vi "Periodic Step Down.vi"(8 "error in (no error)":errorcluster caption="entrée d'erreur (pas d'erreur)", 11 "Game Board en entrée":refnum<class "Game Board.lvclass">) -> (0 "error out":errorcluster caption="sortie d'erreur", 2 "Freeze Piece":bool, 3 "Game Board en sortie":refnum<class "Game Board.lvclass">)   [LabVIEW 2017, in "Game Board.lvclass"]
uses:
  Game Board.lvclass
  Controls/Moves.ctl
  Controls/Coordinates.ctl
  Game Board.lvclass/Game Board.ctl
  Piece of Bricks_class/Piece of Bricks.lvclass
  Wall_class/Wall.lvclass
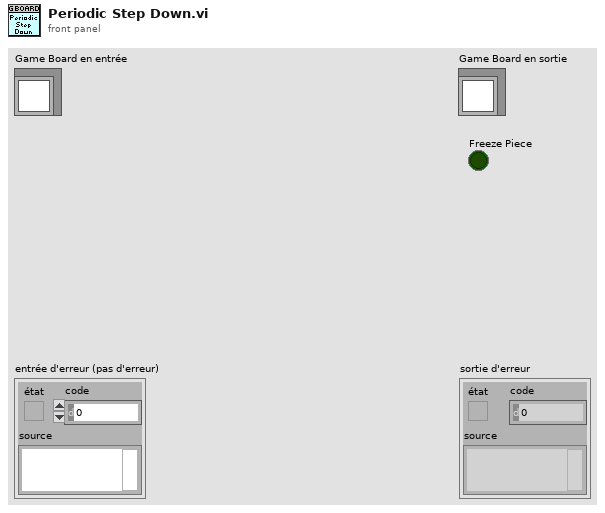
[diagram p1: front panel]
types:
  T1 = typedef "Coordinates.ctl" = cluster{"X":i32, "Y":i32}
  T2 = typedef "Moves.ctl" = enum16{"None", "Right", "Left", "Step Down", "Go Down", "90 Clockwise", "90 Anti-Clockwise"}
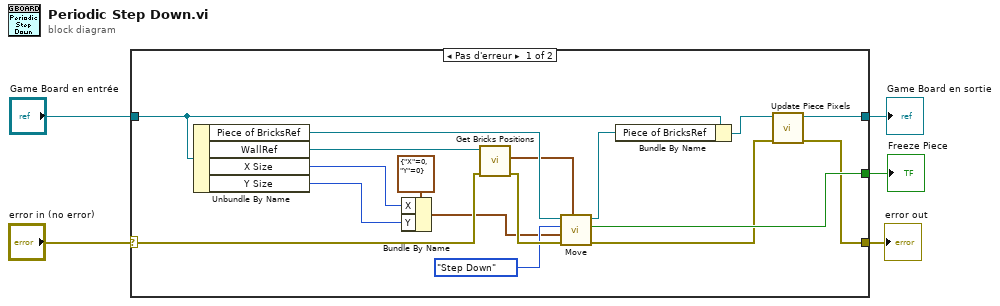
[diagram p0: block diagram]
diagram:
  n1 = case shown="Pas d'erreur" "error in (no error)" {
    selector: "error in (no error)" -> [w22 w24]
    tunnel: [w8 w24] -> w4
    tunnel: [w10 w23] -> w2
    tunnel: "Game Board en entrée" -> [w21 w23]
    tunnel: [w12 _] -> w1
    frame No Error {
      n2 = Unbundle By Name(w21) -> ("Piece of BricksRef"=w20:refnum<class "Piece of Bricks.lvclass">, "WallRef"=w18:refnum<class "Wall.lvclass">, "X Size"=w7:i32, "Y Size"=w6:i32)
      n3 = Bundle By Name(cluster=T1 {"X"=0, "Y"=0} ("Coordinates"), "X"=w7, "Y"=w6) -> (w13:T1)
      n4 = call-dynamic "Get Bricks Positions.vi"("error in (no error)"=w22, "object in"=w18) -> ("error out"=w16:errorcluster, "Brick Wall"=w17:T1[])  [unwired: 7 in, 1 out]
      n5 = call-dynamic "Move.vi"("Wall Positions"=w17, "error in (no error)"=w16, "GameBoard Size"=w13, "Move"=Moves."Step Down", "object in"=w20) -> ("error out"=w9:errorcluster, "Freeze Piece"=w12:bool, "object out"=w19:refnum<class "Piece of Bricks.lvclass">)  [unwired: 4 in]
      n6 = Bundle By Name(cluster=w21, "Piece of BricksRef"=w19) -> (w11:refnum<class "Game Board.lvclass">)
      n7 = call-dynamic "Update Piece Pixels.vi"("error in (no error)"=w9, "Game Board en entrée"=w11) -> ("error out"=w8:errorcluster, "Game Board en sortie"=w10:refnum<class "Game Board.lvclass">)  [unwired: 8 in]
    }
    frame Error {
    }
  }
  "error out" <- w4
  "Game Board en sortie" <- w2
  "Freeze Piece" <- w1
